vi "dfd_FLP IIR II Transposed.vi"(7 "x":dbl format="%.2f", 9 "states in":dbl[](array[numeric]) format="%.2f", 10 "coefficients a":dbl[](array[numeric]) format="%.2f", 11 "coefficients b":dbl[](array[numeric]) format="%.2f") -> (1 "states out":dbl[](array[numeric]) format="%.2f", 3 "y":dbl format="%.2f")   [LabVIEW 2017, in "NI_DigFilter_FXP.lvlib"]
uses:
  <vilib>/addons/Digital Filter Design/NI_DigFilter_FXP.lvlib
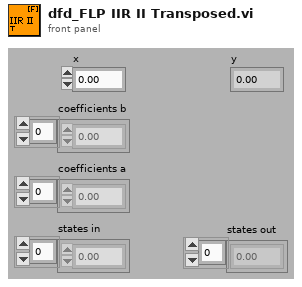
[diagram p1: front panel]
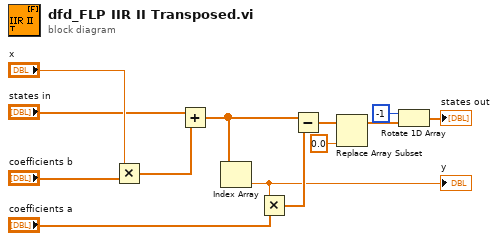
[diagram p0: block diagram]
diagram:
  n1 = Multiply(x="x", y="coefficients b") -> (x*y=w12:dbl[])
  n2 = Add(x="states in", y=w12) -> (x+y=w6:dbl[])
  n3 = Index Array(array=w6) -> (element=w5:dbl)  [unwired: 1 in]
  "y" <- w5
  n4 = Multiply(x=w5, y="coefficients a") -> (x*y=w11:dbl[])
  n5 = Subtract(x=w6, y=w11) -> (x-y=w10:dbl[])
  n6 = Replace Array Subset(array=w10, new element=0.0 ("new element/subarray")) -> (w4:dbl[])  [unwired: 1 in]
  n7 = Rotate 1D Array(1:w4, 2:-1 ("n")) -> (0:→"states out":dbl[])
